vi "Read Thermocouples and Voltages v190401_A.vi"() -> ()   [LabVIEW 2017]
doc: "I. Description:\nThis example demonstrates how to make continuous, hardware-timed temperature measurement using a thermocouple.\n\nII. Instructions for Running:\n1. Specify the Physical Channel where you have connected the thermocouple.\n2. Enter the Minimum and Maximum temperature values in degrees C you expect to measure. A smaller range will allow a more accurate measurement.\n3. Enter the scan rate at which you want to run the acquisition.\n4. Specify the type of thermocouple you are using.\n5. Thermocouple measurements require cold-junction compensation (CJC) to correctly scale them. Specify the source of your cold-junction compensation.\n6. If your CJC source is \"Internal\", skip the rest of the steps.\n7. If your CJC source is \"Constant Value\", specify the value (usually room temperature) in degrees C.\n8. If your CJC source is \"Channel\", specify the CJC Channel name. \n9. Specify the appropriate Auto Zero Mode. See your device's hardware manual to find out if your device supports this attribute.\n\nIII. Block Diagram Steps:\n1. Create a Thermocouple (TC) temperature measurement channel.\n2. Get all the channels in the task.\n3. Convert channel(s) array to a comma-delimited channel string.\n4. This attribute is set to compensate for input offset errors. May not be supported by all devices*.\n5. Call the Timing VI to specify the hardware timing parameters. Use device's internal clock, continuous mode acquisition and the sample rate specified by the user.\n6. Call the Start VI to program and start the acquisition.\n7. Read N samples and plot it. By default, the Read VI reads all available samples, but you can specify how many samples to read at a time and the timeout value. Continue reading data until the stop button is pressed or an error occurs. \n8. Call the Clear Task VI to clear the Task.\n9. Use the popup dialog box to display an error if any.\n\n* If your device does not support Auto Zero Mode bypass Step 2, 3, and 4.\n\nIV. I/O Connections Overview:\nConnect your thermocouple to the terminals corresponding to the Physical Channel I/O Control value."
uses:
  <vilib>/Utility/error.llb/DialogType.ctl
  <vilib>/DAQmx/write.llb/DAQmx Write (Digital 1D Bool NChan 1Samp 1Line).vi
  <vilib>/DAQmx/read.llb/DAQmx Read (Analog 1D Wfm NChan NSamp).vi
  <vilib>/Analysis/baseanly.llb/Mean (DBL).vi
  <vilib>/DAQmx/create/channels.llb/DAQmx Create Channel (DO-Digital Output).vi
  <vilib>/Waveform/WDTOps.llb/WDT Index Channel DBL.vi
  <vilib>/DAQmx/create/channels.llb/DAQmx Create Channel (AI-Voltage-Basic).vi
  <vilib>/DAQmx/configure/timing.llb/DAQmx Timing (Sample Clock).vi
  <vilib>/DAQmx/miscellaneous.llb/DAQmx Fill In Error Info.vi
  <vilib>/express/express arith-compare/Formula/XNode/ExpressFormulaBlockNode.xnode
  <vilib>/Analysis/NI_AALBase.lvlib
  <vilib>/ptbypt/NI_PtbyPt.lvlib
  <vilib>/Utility/miscctls.llb/LVRowAndColumnTypeDef.ctl
panel:
  in  "Color Box":u32(colorbox)=16448250
  out "Micro-strain":dbl[](array[numeric]) format="%.2g"
  out "Results":i32[](listbox)
  in  "num_chans":i32=32
  in  "Search Strings":string[](array[string])=["Verbose Name", "Units", "Sensitivity", "Offset"]
  out "TRQ_2SPD_OT (N·m)":dbl=-0.01305389404296875 format="%0.3f"
  out "Power_OT (W)":dbl=-4.779110606064606 format="%.2f"
  out "rpm_out/rpm_in":dbl=-8.382425226893735e-05 format="%.3g"
  out "switch_counts":dbl=4500000.0
  in  "switch_time (s)":dbl=900000.0
  out "AI Consumer Iterations":i32=391128
  in  "LV_CMD_2SPD_OIL_SLND":bool[](array[boolean])=[FALSE]
  in  "lines":tag="Dev3/port1/line0"
  out "RPM_2SPD_OT_6602":dbl format="%0.1f"
  in  "path":path=path "N:/TeamShares/Testing Group/Bench Tests/PR22965 - Flow Test Magnum Lube Components/LabView Data"
  in  "DRVLN_PULLEY_RATIO":dbl=1.48 format="%.2f"
  out "P2 - P1":dbl=2.2560862731933593 format="%.3f"
  out "Recorded Blocks":dbl=295196.0
  out "AI Producer Iterations":i32=391127
  in  "Force Record":bool caption="Force Record Enable"
  out "RPM_DRVLN_6602":dbl format="%0.1f"
  out "data 2":waveform(dbl)[](array[waveform])=[{"t0"=timestamp(3621510319.1461306 s since 1904-01-01), "dt"=0.1, "Y"=[-0.0004730224609375, 0.00026397705078125], "attributes"=variant("NI_ChannelName"=variant(string "Dev1/ai0"), "NI_UnitDescription"=variant(string "Volts"))}, {"t0"=timestamp(3621510319.1461306 s since 1904-01-01), "dt"=0.1, "Y"=[1.0218643188476562, 1.0218521118164063], "attributes"=variant("NI_ChannelName"=variant(string "Dev1/ai0"), "NI_UnitDescription"=variant(string "Volts"))}, {"t0"=timestamp(3621510319.1461306 s since 1904-01-01), "dt"=0.1, "Y"=[1.5897842407226563, 1.5984542846679688], "attributes"=variant("NI_ChannelName"=variant(string "Dev1/ai0"), "NI_UnitDescription"=variant(string "Volts"))}, {"t0"=timestamp(3621510319.1461306 s since 1904-01-01), "dt"=0.1, "Y"=[1.525469970703125, 1.533917236328125], "attributes"=variant("NI_ChannelName"=variant(string "Dev1/ai0"), "NI_UnitDescription"=variant(string "Volts"))}, {"t0"=timestamp(3621510319.1461306 s since 1904-01-01), "dt"=0.1, "Y"=[3.0046722412109377, 3.0046966552734373], "attributes"=variant("NI_ChannelName"=variant(string "Dev1/ai0"), "NI_UnitDescription"=variant(string "Volts"))}, {"t0"=timestamp(3621510319.1461306 s since 1904-01-01), "dt"=0.1, "Y"=[1.769482421875, 1.7677413940429687], "attributes"=variant("NI_ChannelName"=variant(string "Dev1/ai0"), "NI_UnitDescription"=variant(string "Volts"))}, {"t0"=timestamp(3621510319.1461306 s since 1904-01-01), "dt"=0.1, "Y"=[-0.0179168701171875, -0.0179443359375], "attributes"=variant("NI_ChannelName"=variant(string "Dev1/ai0"), "NI_UnitDescription"=variant(string "Volts"))}, {"t0"=timestamp(3621510319.1461306 s since 1904-01-01), "dt"=0.1, "Y"=[-0.0014312744140625, -0.00116424560546875], "attributes"=variant("NI_ChannelName"=variant(string "Dev1/ai0"), "NI_UnitDescription"=variant(string "Volts"))}, {"t0"=timestamp(3621510319.1461306 s since 1904-01-01), "dt"=0.1, "Y"=[-0.00082550048828125, -0.0017852783203125], "attributes"=variant("NI_ChannelName"=variant(string "Dev1/ai0"), "NI_UnitDescription"=variant(string "Volts"))}, {"t0"=timestamp(3621510319.1461306 s since 1904-01-01), "dt"=0.1, "Y"=[2.997636413574219, 2.9961593627929686], "attributes"=variant("NI_ChannelName"=variant(string "Dev1/ai0"), "NI_UnitDescription"=variant(string "Volts"))}, {"t0"=timestamp(3621510319.1461306 s since 1904-01-01), "dt"=0.1, "Y"=[-1.52587890625e-05, -0.00017242431640625], "attributes"=variant("NI_ChannelName"=variant(string "Dev1/ai0"), "NI_UnitDescription"=variant(string "Volts"))}, {"t0"=timestamp(3621510319.1461306 s since 1904-01-01), "dt"=0.1, "Y"=[0.002484130859375, 0.00252532958984375], "attributes"=variant("NI_ChannelName"=variant(string "Dev1/ai0"), "NI_UnitDescription"=variant(string "Volts"))}, {"t0"=timestamp(3621510319.1461306 s since 1904-01-01), "dt"=0.1, "Y"=[-0.10861358642578126, -0.10858306884765626], "attributes"=variant("NI_ChannelName"=variant(string "Dev1/ai0"), "NI_UnitDescription"=variant(string "Volts"))}, {"t0"=timestamp(3621510319.1461306 s since 1904-01-01), "dt"=0.1, "Y"=[-1.1660736083984375, -1.1659881591796875], "attributes"=variant("NI_ChannelName"=variant(string "Dev1/ai0"), "NI_UnitDescription"=variant(string "Volts"))}, {"t0"=timestamp(3621510319.1461306 s since 1904-01-01), "dt"=0.1, "Y"=[-1.0824356079101562, -1.0823379516601563], "attributes"=variant("NI_ChannelName"=variant(string "Dev1/ai0"), "NI_UnitDescription"=variant(string "Volts"))}, {"t0"=timestamp(3621510319.1461306 s since 1904-01-01), "dt"=0.1, "Y"=[-0.1474090576171875, -0.14737548828125], "attributes"=variant("NI_ChannelName"=variant(string "Dev1/ai0"), "NI_UnitDescription"=variant(string "Volts"))}]
  out "Power_IN (W)":dbl=0.0005711775684961294 format="%.2g"
  out "TRQ_2SPD_DRVLN_OT (N·m)":dbl=-0.018612060546874976 format="%0.3f"
  out "Waveform Chart":waveform(dbl)[](graph)=[{"t0"=timestamp(3634059218.103555 s since 1904-01-01), "dt"=0.1, "Y"=[0.0040825469970704464, 0.004508938598632994], "attributes"=variant("NI_ChannelName"=variant(string "P1_OIL_FILTER_OT"), "NI_UnitDescription"=variant(string "bar g"))}, {"t0"=timestamp(3634059218.103555 s since 1904-01-01), "dt"=0.1, "Y"=[2.0849262466430662, 2.0811629058837893], "attributes"=variant("NI_ChannelName"=variant(string "P2_OIL_PUMP_CTRL"), "NI_UnitDescription"=variant(string "bar g"))}, {"t0"=timestamp(3634059218.103555 s since 1904-01-01), "dt"=0.1, "Y"=[2.0002626892089843, 1.9966154815673829], "attributes"=variant("NI_ChannelName"=variant(string "P3_OIL_PUMP_OT"), "NI_UnitDescription"=variant(string "bar g"))}, {"t0"=timestamp(3634059218.103555 s since 1904-01-01), "dt"=0.1, "Y"=[-11.107454470825196, -11.112982447814943], "attributes"=variant("NI_ChannelName"=variant(string "P4_OIL_LUBE_OT"), "NI_UnitDescription"=variant(string "bar g"))}, {"t0"=timestamp(3634059218.103555 s since 1904-01-01), "dt"=0.1, "Y"=[-2.105040821838379, -2.1068857055664063], "attributes"=variant("NI_ChannelName"=variant(string "P5_SPARE"), "NI_UnitDescription"=variant(string "bar g"))}, {"t0"=timestamp(3634059218.103555 s since 1904-01-01), "dt"=0.1, "Y"=[-3.1523495605468748, -3.15418076171875], "attributes"=variant("NI_ChannelName"=variant(string "P6_SPARE"), "NI_UnitDescription"=variant(string "bar g"))}, {"t0"=timestamp(3634059218.103555 s since 1904-01-01), "dt"=0.1, "Y"=[-0.927960205078125, -0.9276962280273438], "attributes"=variant("NI_ChannelName"=variant(string "P7_SPARE"), "NI_UnitDescription"=variant(string "bar a"))}, {"t0"=timestamp(3634059218.103555 s since 1904-01-01), "dt"=0.1, "Y"=[0.02285817565917947, 0.02207293701171853], "attributes"=variant("NI_ChannelName"=variant(string "P8_OIL_COOLER_OT"), "NI_UnitDescription"=variant(string "bar g"))}, {"t0"=timestamp(3634059218.103555 s since 1904-01-01), "dt"=0.1, "Y"=[1410.0847681655885, 1409.1728451538086], "attributes"=variant("NI_ChannelName"=variant(string "RPM_2SPD_IN_FV"), "NI_UnitDescription"=variant(string "RPM"))}, {"t0"=timestamp(3634059218.103555 s since 1904-01-01), "dt"=0.1, "Y"=[1374.9208407257079, 1374.7411578094482], "attributes"=variant("NI_ChannelName"=variant(string "RPM_2SPD_OT_FV"), "NI_UnitDescription"=variant(string "RPM"))}, {"t0"=timestamp(3634059218.103555 s since 1904-01-01), "dt"=0.1, "Y"=[51.3275146484375, 51.390533447265625], "attributes"=variant("NI_ChannelName"=variant(string "T_OIL_PUMP_OT"), "NI_UnitDescription"=variant(string "°C"))}, {"t0"=timestamp(3634059218.103555 s since 1904-01-01), "dt"=0.1, "Y"=[69.04945373535156, 69.14482116699219], "attributes"=variant("NI_ChannelName"=variant(string "T_OIL_SPARE"), "NI_UnitDescription"=variant(string "°C"))}, {"t0"=timestamp(3634059218.103555 s since 1904-01-01), "dt"=0.1, "Y"=[-4.136749267578125, -4.28717041015625], "attributes"=variant("NI_ChannelName"=variant(string "TRQ_PMP_IN"), "NI_UnitDescription"=variant(string "N·m"))}, {"t0"=timestamp(3634059218.103555 s since 1904-01-01), "dt"=0.1, "Y"=[-0.009429931640625, -0.0040740966796875], "attributes"=variant("NI_ChannelName"=variant(string "TRQ_2SPD_OT"), "NI_UnitDescription"=variant(string "N·m"))}, {"t0"=timestamp(3634059218.103555 s since 1904-01-01), "dt"=0.1, "Y"=[0.22497978210449232, 0.2247674942016602], "attributes"=variant("NI_ChannelName"=variant(string "VFr_660_0380_OT"), "NI_UnitDescription"=variant(string "gpm"))}, {"t0"=timestamp(3634059218.103555 s since 1904-01-01), "dt"=0.1, "Y"=[-14.992698669433594, -14.993682861328125], "attributes"=variant("NI_ChannelName"=variant(string "VFr_OIL_LUBE_OT"), "NI_UnitDescription"=variant(string "gpm"))}, {"t0"=timestamp(3634059218.103555 s since 1904-01-01), "dt"=0.1, "Y"=[1.48, 1.48], "attributes"=variant("NI_ChannelName"=variant(string "RPM_RATIO"), "NI_UnitDescription"=variant(string "ratio"))}, {"t0"=timestamp(3634059218.103555 s since 1904-01-01), "dt"=0.1, "Y"=[99.0, 99.0], "attributes"=variant("NI_ChannelName"=variant(string "DataTag"), "NI_UnitDescription"=variant(string "none"))}, {"t0"=timestamp(3634059218.103555 s since 1904-01-01), "dt"=0.1, "Y"=[0.0, 0.0], "attributes"=variant("NI_ChannelName"=variant(string "LV_CMD_2SPD_OIL_SLND"), "NI_UnitDescription"=variant(string "boolean"))}]
  in  "Run Letter":string="a"
  out "Recording":bool
  in  "Num_Blocks":dbl=100.0
  in  "Data Tag":dbl=99.0 format="%.2p"
  in  "Maximum Value":dbl=10.0 format="%0.2f"
  in  "Minimum Value":dbl=-10.0 format="%0.2f"
  in  "Physical Channel":tag="Dev4/ai0:31" caption="PCI-6143_1 Channels"
  in  "stop":bool
  in  "Rate":dbl=1000.0 format="%0.2f"
  # "rev 150415_A  added \"Record Run X\" sub VI.\nrev 150423_A added power, efficiency, and manual inputs for speed .\nrev 150423_B added speed measurement via PCI-6602 card.\nrev 161117_A is set up for the alternator test reading shaft RPM from Dynapar encoder and torque from the Omega TQ513-1K paired with the Omega DP41-S.\nrev 170504_A migrated DAQ h/w from the SCXI chassis (now being used for TC2 porcupine testing) to PCI-6143.\nrev 170510_A takes data at 1000Hz, then averages groups of 100 samples for a logging rate of 10Hz per channel.  Added function that resets \"Data Tag\"\nto 99 after \"Num_Blocks\" has been recorded.\nrev 170810_A adds flowmeter for 2-speed supercharger drive bench test.  CJP\nrev 170821_A logs tags to same file for a given run letter.  Uses \"Record Continuous Tags...\" sub VI.\nrev 171129_A is for the Orthrus 2-speed drive.  Added new encoder period measurement for the 127 tooth geat \"RPM_2SPD_OT\". CJP\nrev 171130_A adds Digital Output (DO) for 2SPD drive control.  Will log this with the rest of the data.  Also corrected the number of teeth on the 2SPD Output side from 127 to 107!\nrev 171201_A restructuring for  \"real-time\" response to speed changes by moving the disklog to a separate loop (queue).\nrev 171201_B moves counters into main AI loop and adds a start trigger so DAQ won't start until rig is spinning.  Added F-V where old \"F1\" channel was for \"RPM_2SPD_OT\".   CJP\nrev 171201_C uses a CI-Frequency task for RPM instead of period.  Testing this for better transient response.  This appears to be even slower than the period measurement.\nrev 171201_D is built from rev 171201_A, but adding in the F-V channel.  This version queues both the AI channel and CI channels to a single Consumer.  Also adding a 30s switch to automate switching of the 2SPD solenoid.\nrev 171221_A was the first attempt at this and for some reason, while running that VI, the computer froze, unable to do ctrl+alt+del reboot.  After rebooting, the VI was no longer openable in LabView 2014 or LabView 2016.  Will try the same process over with v171226_A.\nrev 171226_A adds one more PCI_6143 card for 8 additional analog inputs.\nrev 171226_B created a backup with 171226_A.\nrev 180314_A added thermocouple for Sumanth.  This is for testing the 2-Speed Drive.\nrev Read \"ThermVolt_TestSpeed_180406_A.vi\" is for verifying the one remaining Micro-Epsilon speed sensor on the 2Spd Drive.\nrev \"Read Thermocouples and Voltages v180406_A.vi\" reintroduces the two counter/timer channels on the PCI-6602 card for the driveline encoder and \nMicro-Epsilon 2Spd Output.\nrev 180919_A built off of rev 180426_A for 2-Speed Drive testing.  CJP\nv181002_A adding new T22 at 2SPD input pulley AND keeping original T22 at output end of drivline.  CJP\nv181004_A corrected front panel displays for Power_IN and Power_OT.  CJP\nv181025_A adding ReadChnCfg.VI to read channel names, units, scaling, and offset from Labview Channel Map\nv190401_A restructuring \"Read Thermocouples and Voltages...\" to use only channels from NI-6229 out of test cell 2.  CJP"
  # "For instructions, select Help>>Show Context Help"
  # "Now using 360 PPR encoder for input speed 171227.\nChanged to Input Gear Speed 180118.  CJP  127 Hz = 1 RPS, 127 Hz = 60 RPM\n5 kHz = 1 V => 5000/127 = 39.37 RPS = 2362.205 RPM\nv180314_A 5kHz = 1V = 5000/360 = 13.888 RPS = 833.33 RPM.\nBack to 360PPR encoder with pulley ratio of 1.48."
  # "HBM T21WN"
  # "Interface T22"
  # "Timing Parameters"
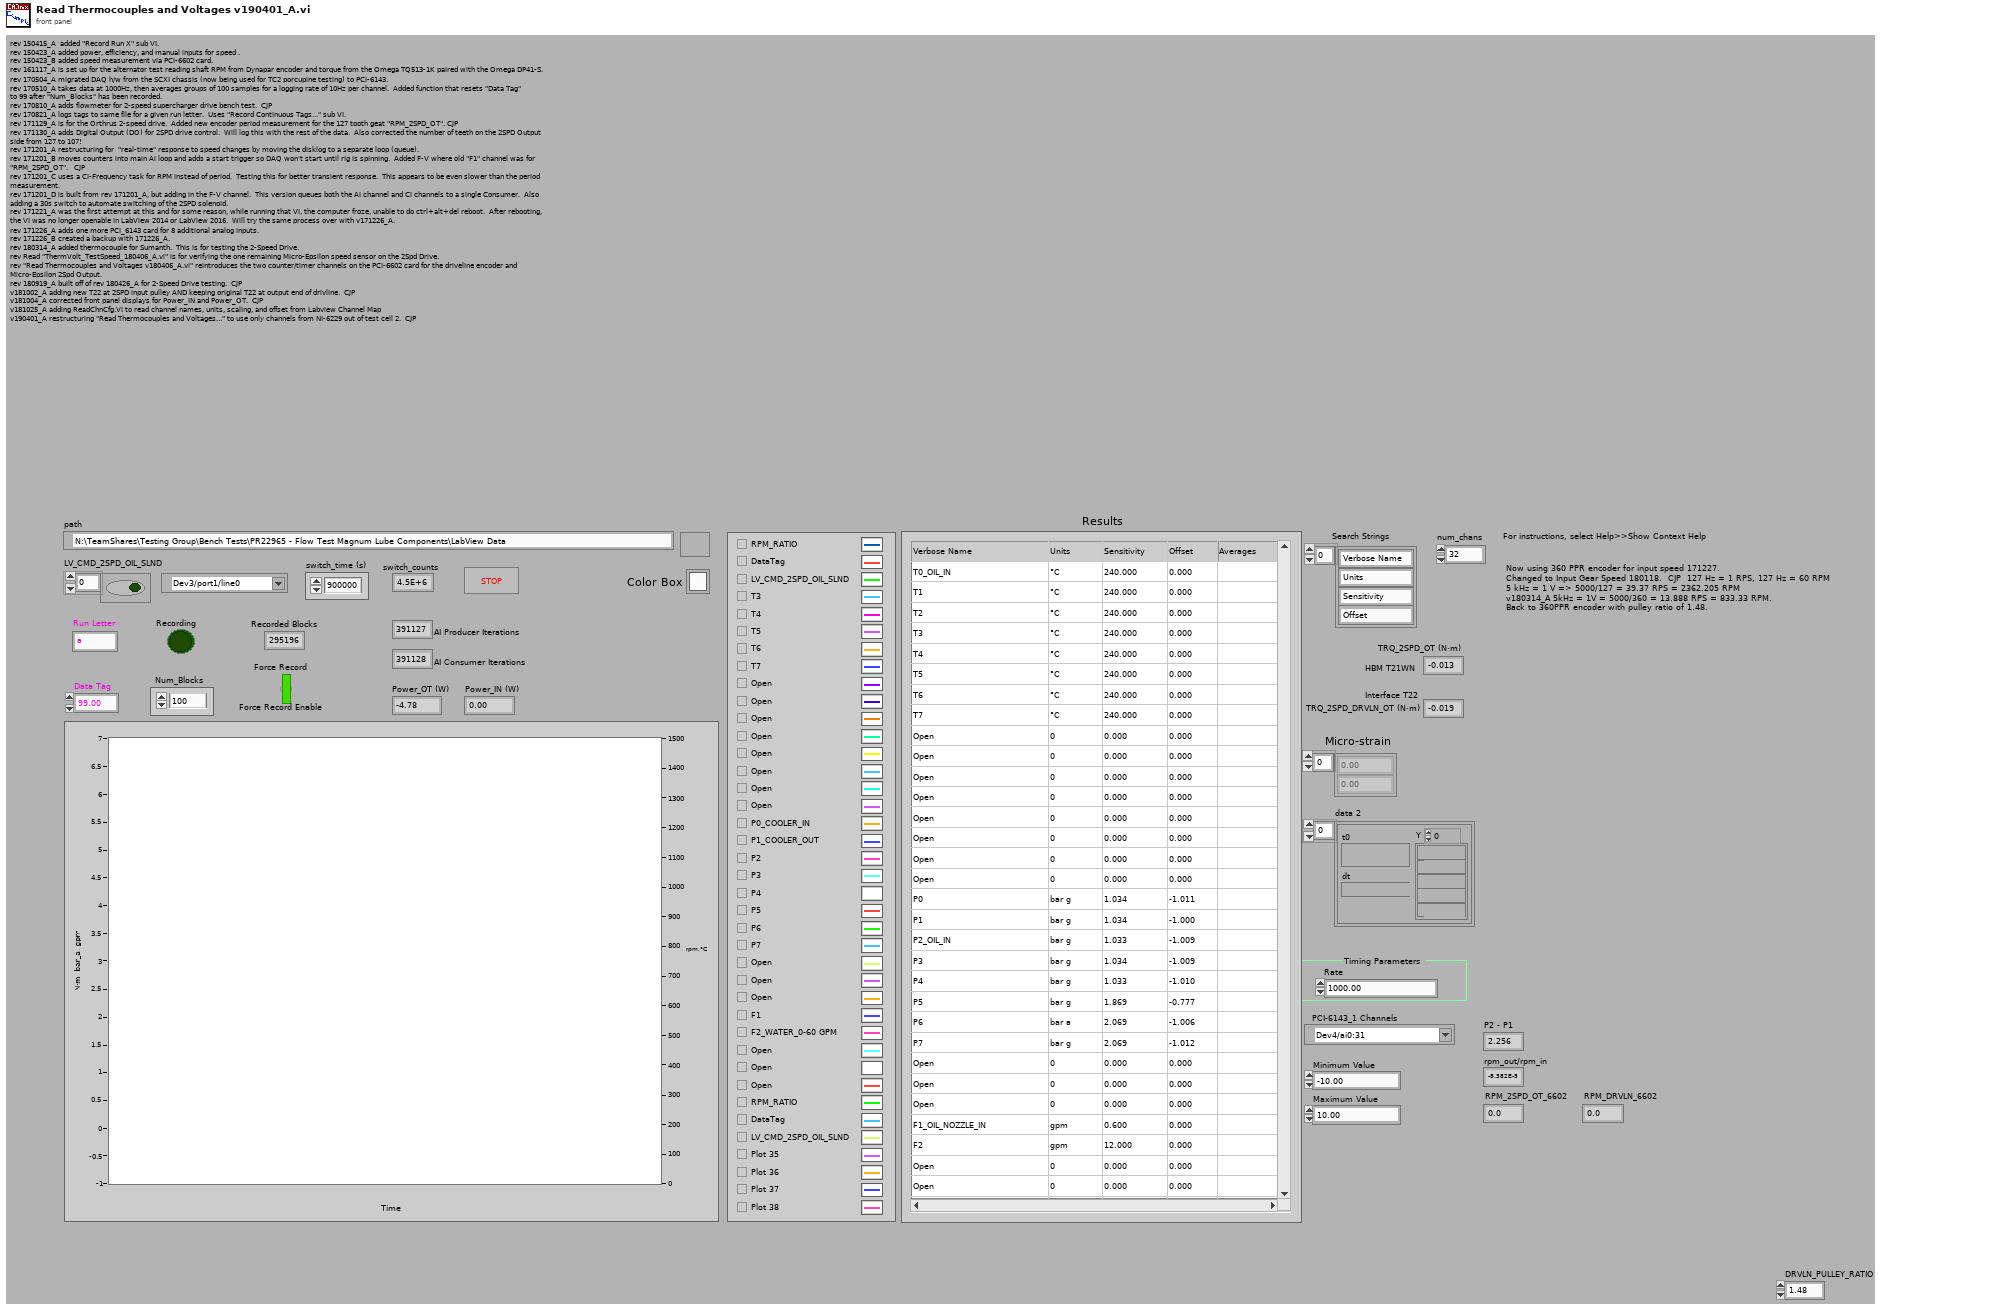
[diagram p1: front panel]
types:
  T1 = typedef "DialogType.ctl" = u16
  T2 = typedef "LVRowAndColumnTypeDef.ctl" = cluster{"Row":i32, "Column":i32}
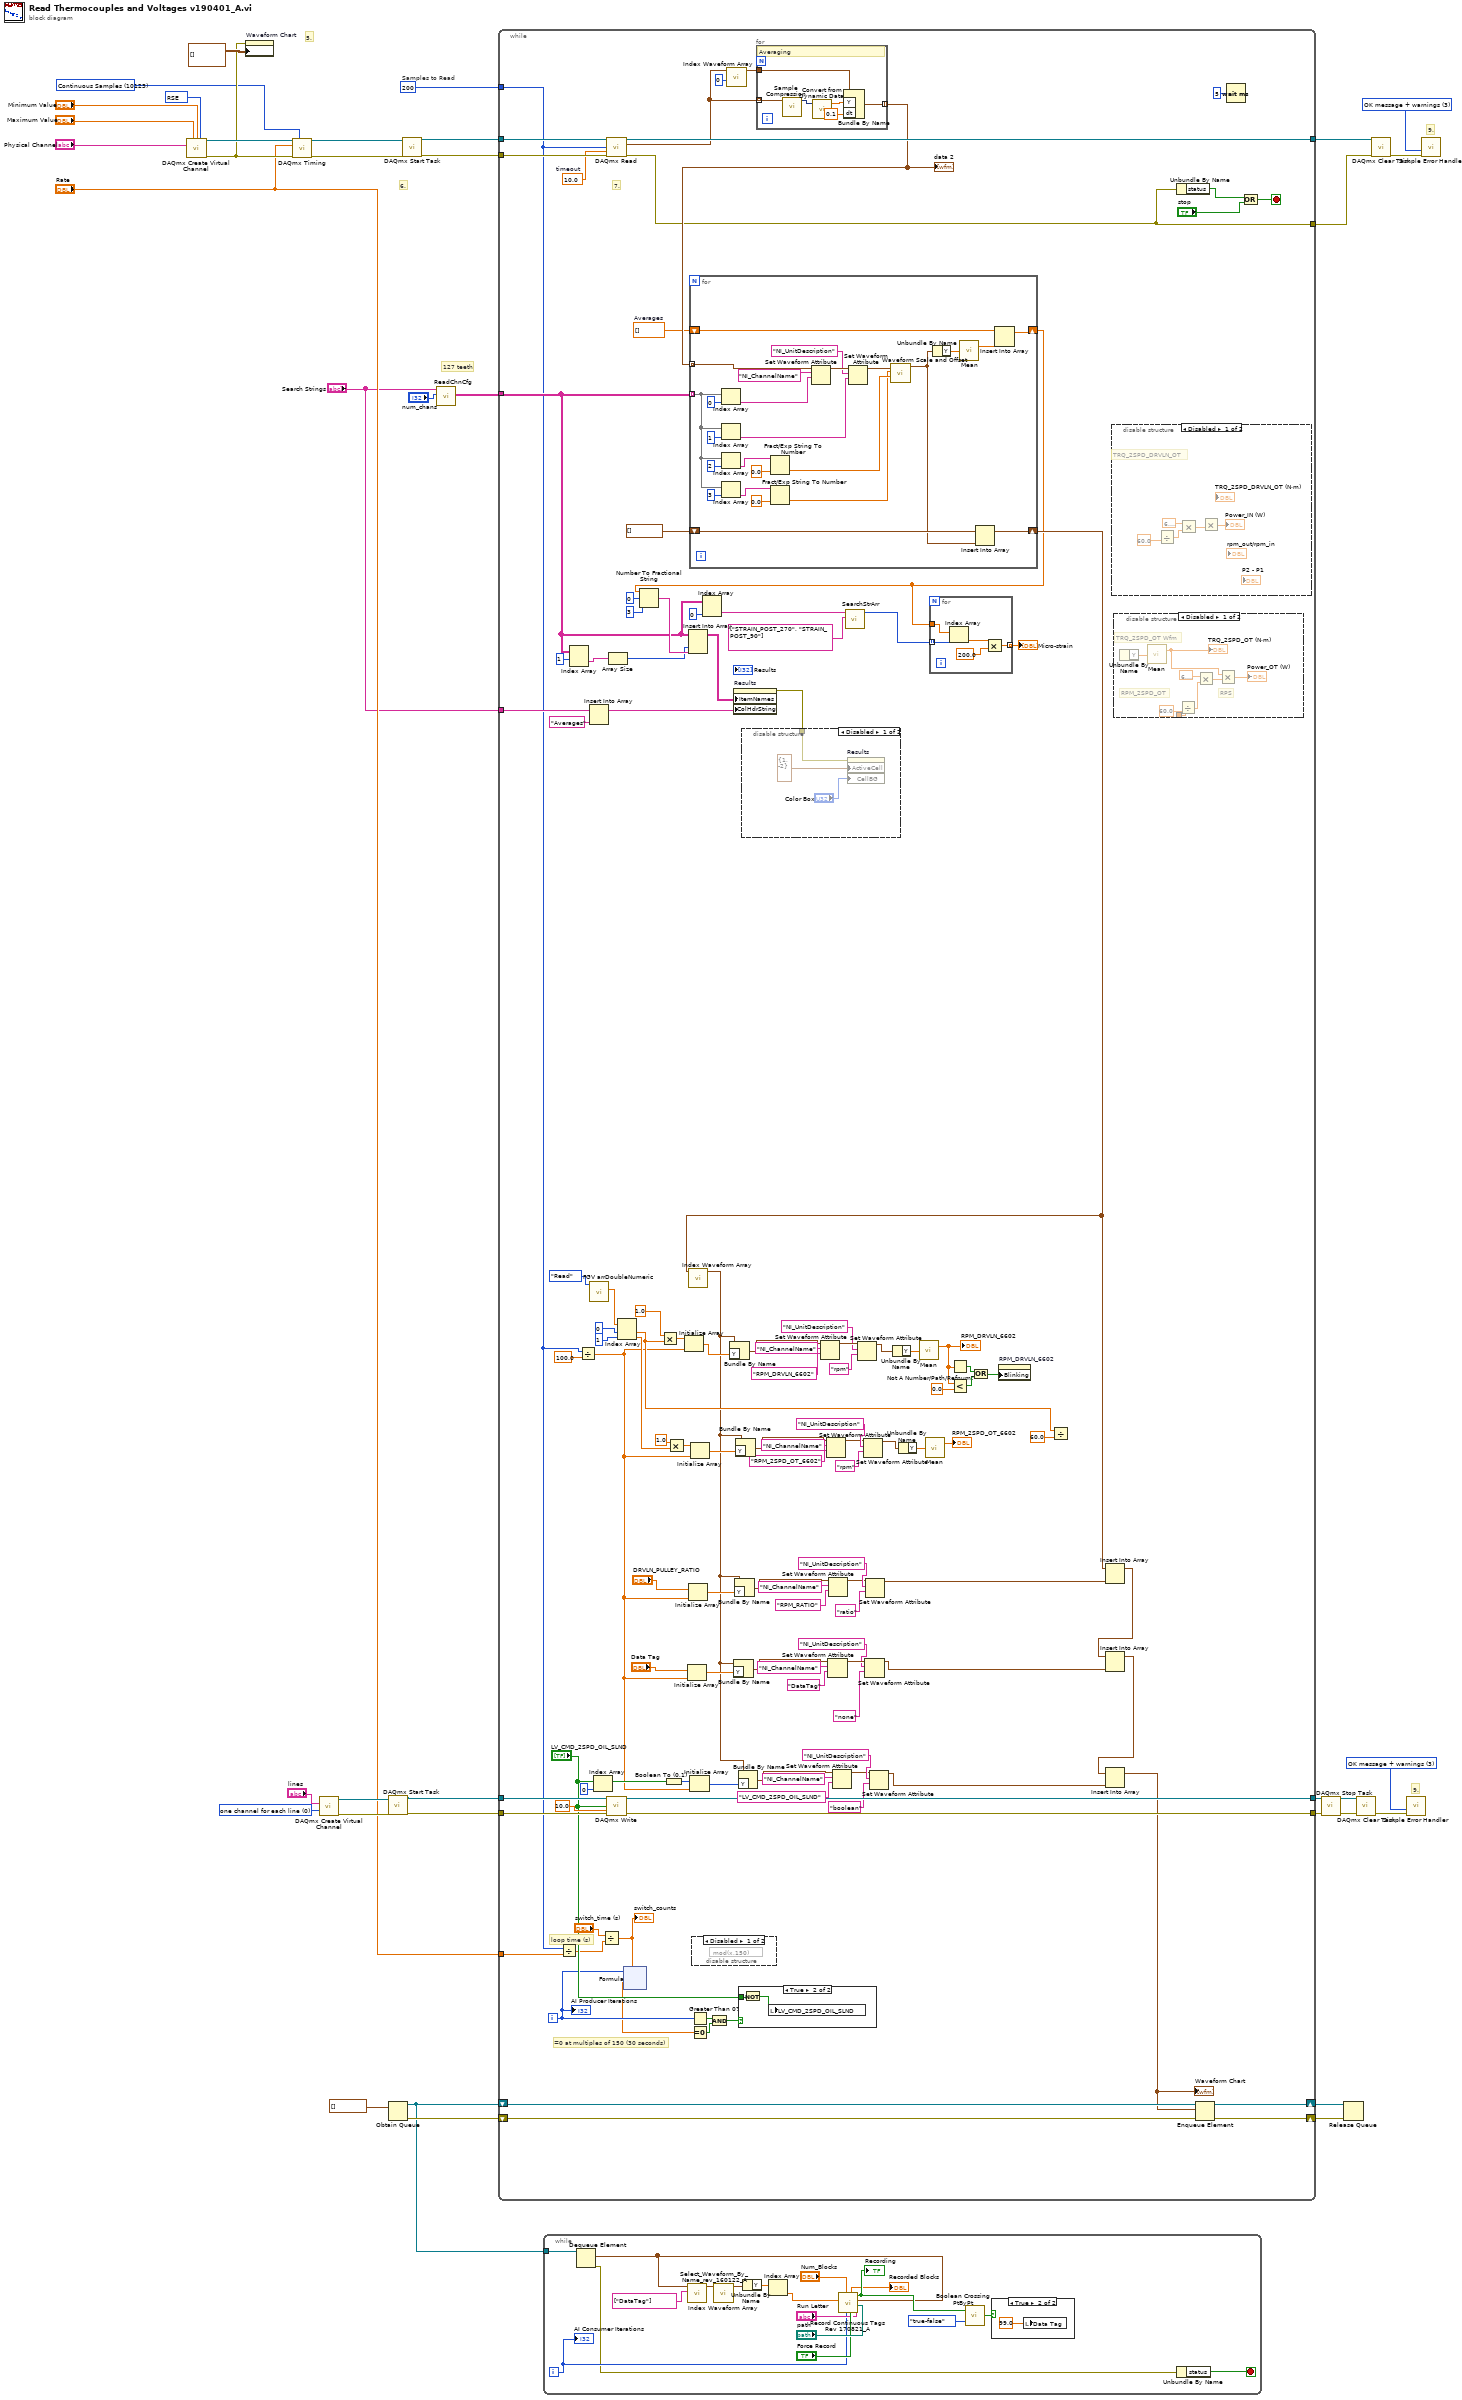
[diagram p0: block diagram]
diagram:
  w1 = 10083 items=["Default"=-1, "RSE"=10083, "NRSE"=10078, "Differential"=10106, "Pseudodifferential"=12529] ("input terminal configuration")
  w21 = T1 3 items=["no dialog", "OK message", "continue or stop message", "OK message + warnings", "continue/stop + warnings"] ("type of dialog (OK msg:1)")
  w27 = 0 items=["one channel for each line", "one channel for all lines"] ("line grouping")
  w33 = T1 3 items=["no dialog", "OK message", "continue or stop message", "OK message + warnings", "continue/stop + warnings"] ("type of dialog (OK msg:1)")
  w7 = 10123 items=["Finite Samples"=10178, "Continuous Samples"=10123] ("sample mode")
  # "127 teeth"
  # "Samples to Read"
  # "9."
  # "9."
  # "5."
  # "6."
  n1 = call-poly <vilib>:"DAQmx Create Virtual Channel.vi"("maximum value"="Maximum Value", "minimum value"="Minimum Value", "input terminal configuration"=w1, "physical channels"="Physical Channel") -> ("task out"=w31:refnum<k21>, "error out"=w29:errorcluster)  [unwired: 10 in]
  n2 = property on="Waveform Chart" class="WFChart (strict)"(error in=w29, "History Data"=waveform(dbl)[][] []) -> ()  [unwired: 1 in, 2 out]
  n3 = call-poly <vilib>:"DAQmx Timing.vi"("task/channels in"=w31, "sample mode"=w7, "rate"="Rate", "error in"=w29) -> ("task out"=w34:refnum<k21>, "error out"=w2:errorcluster)  [unwired: 10 in]
  n4 = call-poly <vilib>:"DAQmx Create Virtual Channel.vi"("lines"="lines", "line grouping"=w27) -> ("task out"=w26:refnum<k21>, "error out"=w25:errorcluster)  [unwired: 12 in]
  n5 = call <vilib>:"DAQmx Start Task.vi"("task/channels in"=w26, "error in"=w25) -> ("task out"=w24:refnum<k21>, "error out"=w23:errorcluster)  [unwired: 12 in]
  n6 = Obtain Queue(element data type=waveform(dbl)[] [] ("appended array")) -> (queue out=w11:refnum<queue>, error out=w14:errorcluster)  [unwired: 4 in, 1 out]
  n7 = call <vilib>:"DAQmx Start Task.vi"("task/channels in"=w34, "error in"=w2) -> ("task out"=w36:refnum<k21>, "error out"=w37:errorcluster)  [unwired: 12 in]
  n8 = call "ReadChnCfg.vi"("num_chans"="num_chans", "Search Strings"="Search Strings") -> ("Table Minus Headers"=w5:string[][])  [unwired: 8 in, 1 out]
  n9 = while {
    tunnel: w36 -> [w162]
    tunnel: w37 -> [w161]
    tunnel: [w160] -> w35
    tunnel: 200 ("number of samples per channel") -> [w40]
    tunnel: w24 -> [w106]
    tunnel: w23 -> [w105]
    tunnel: [w104] -> w18
    tunnel: [w103] -> w17
    shift-right: [w89] -> w13
    shift-left: w11 -> [w91]
    shift-right: [w88] -> w12
    shift-left: w14 -> [w90]
    tunnel: "Rate" -> [w82]
    tunnel: [w42] -> w3
    tunnel: w5 -> [w49]
    tunnel: "Search Strings" -> [w59]
    i -> [w79]
    stop <- w157 stop-if-true
    w70 = dbl[] []  # Averages
    w158 = 10.0  # timeout
    # "loop time (s)"
    # "=0 at multiples of 150 (30 seconds)"
    # "7."
    n10 = Divide(x=w40, y=w82) -> (x/y=w81:dbl)
    n11 = Index Array(array=w49, index (row)=1) -> (element=w53:string[])  [unwired: 1 in]
    n12 = Divide(x=w40, y=100.0) -> (x/y=w92:dbl)
    n13 = Insert Into Array(array=w59, new element="Averages" ("new element/subarray")) -> (w50:string[])  [unwired: 1 in]
    n14 = call "FGV arrDoubleNumeric.vi"("Enum"=enum16{"Read", "Write"}."Read") -> ("Array OUT"=w121:dbl[])  [unwired: 9 in, 1 out]
    n15 = Index Array(array="LV_CMD_2SPD_OIL_SLND", index=0) -> (element=w100:bool)
    n16 = Divide(x="switch_time (s)", y=w81) -> (x/y=w78:dbl)
    "switch_counts" <- w78
    n17 = call-poly <vilib>:"DAQmx Read.vi"("task/channels in"=w162, "number of samples per channel"=w40, "timeout"=w158, "error in"=w161) -> ("task out"=w160:refnum<k21>, "data"=w41:waveform(dbl)[], "error out"=w42:errorcluster)  [unwired: 9 in]
    n18 = call-poly <vilib>:"DAQmx Write.vi"("task/channels in"=w106, "data"="LV_CMD_2SPD_OIL_SLND", "timeout"=10.0, "error in"=w105) -> ("task out"=w104:refnum<k21>, "error out"=w103:errorcluster)  [unwired: 9 in, 1 out]
    n19 = Array Size(array=w53) -> (size(s)=w52:i32)
    n20 = Index Array(array=w121, index #1=0 ("index"), index #2=1 ("index")) -> (element #1=w120:dbl, element #2=w107:dbl)
    n21 = xnode "Formula"("X1"=w79, "X2"=w78) -> ("Result"=w77:dbl)  [unwired: 1 in, 1 out]
    n22 = Multiply(x=1.0, y=w120) -> (x*y=w138:dbl)
    n23 = Boolean To (0,1)(Boolean=w100) -> (0, 1=w93:i16)
    n24 = Multiply(x=1.0, y=w107) -> (x*y=w115:dbl)
    n25 = Initialize Array(w138, w92) -> (w146:dbl[])
    n26 = Initialize Array("Data Tag", w92) -> (w123:dbl[])
    n27 = Initialize Array("DRVLN_PULLEY_RATIO", w92) -> (w136:dbl[])
    n28 = Initialize Array(w93, w92) -> (w87:i16[])
    n29 = Initialize Array(w115, w92) -> (w114:dbl[])
    n30 = Greater Than 0?(x=w79) -> (x > 0?=w84:bool)
    n31 = Equal To 0?(x=w77) -> (x = 0?=w83:bool)
    n32 = disable-structure shown="Disabled" {
      frame Disabled {
        n33 = expression code="mod(x,150)"() -> ()  [unwired: 1 in, 1 out]
      }
      frame Enabled {
      }
    }
    n34 = Index Array(array=w49, index (col)=0 ("disabled index (col)")) -> (element=w47:string[])  [unwired: 1 in]
    n35 = And(x=w84, y=w83) -> (x .and. y?=w85:bool)
    n36 = call-poly <vilib>:"Index Waveform Array.vi"("index"=0, "waveform array"=w41) -> ("waveform"=w139:waveform(dbl))  [unwired: 8 in, 1 out]
    n37 = case shown="True" w85 {
      tunnel: "LV_CMD_2SPD_OIL_SLND" -> [_ w220]
      frame False {
      }
      frame True {
        n38 = Not(x=w220) -> (.not. x?=w219:bool[])
        n39 = local write "LV_CMD_2SPD_OIL_SLND"(w219) -> ()
      }
    }
    n40 = for {
      tunnel: w41 -> [w223] mode=indexing
      tunnel: [w222] -> w72 mode=indexing
      tunnel: w139 -> [w221]
      # "Averaging"
      n41 = call "Sample Compression"("Signals"=w223) -> ("Mean"=w224:dynamicdata)  [unwired: 8 in, 2 out]
      n42 = call "Convert from Dynamic Data"("Dynamic Data Type"=w224) -> ("Array"=w226:dbl[])  [unwired: 3 in]
      n43 = Bundle By Name(cluster=w221, "Y"=w226, "dt"=0.1) -> (w222:waveform(dbl))
    }
    "data 2" <- w72
    n44 = for {
      tunnel: w72 -> [w195] mode=indexing
      shift-right: [w194] -> w44
      shift-left: w70 -> [w193]
      tunnel: w49 -> [w182] mode=indexing
      shift-right: [w189] -> w66
      shift-left: waveform(dbl)[] [] -> [w191]
      n45 = Index Array(array=w182, index=0) -> (element=w186:string)
      n46 = Index Array(array=w182, index=1) -> (element=w185:string)
      n47 = Index Array(array=w182, index=2) -> (element=w181:string)
      n48 = Index Array(array=w182, index=3) -> (element=w177:string)
      n49 = Fract/Exp String To Number(string=w181, default (0 dbl)=0.0) -> (number=w179:dbl)  [unwired: 2 in, 1 out]
      n50 = Fract/Exp String To Number(string=w177, default (0 dbl)=0.0) -> (number=w176:dbl)  [unwired: 2 in, 1 out]
      n51 = Set Waveform Attribute(5:w186, 6:"NI_ChannelName" ("name"), 7:w195) -> (3:w199:waveform(dbl))  [unwired: 1 in, 2 out]
      n52 = Set Waveform Attribute(5:w185, 6:"NI_UnitDescription" ("name"), 7:w199) -> (3:w197:waveform(dbl))  [unwired: 1 in, 2 out]
      n53 = call <vilib>:"Waveform Scale and Offset.vi"("scale"=w179, "offset"=w176, "waveform in"=w197) -> ("waveform out"=w190:waveform(dbl))  [unwired: 7 in, 1 out]
      n54 = Unbundle By Name(w190) -> ("Y"=w196:dbl[])
      n55 = call-poly <vilib>:"Mean.vi"("X"=w196) -> ("mean"=w192:dbl)  [unwired: 1 out]
      n56 = Insert Into Array(array=w191, new element=w190) -> (w189:waveform(dbl)[])  [unwired: 1 in]
      n57 = Insert Into Array(array=w193, new element=w192) -> (w194:dbl[])  [unwired: 1 in]
    }
    n58 = Number To Fractional String(number=w44, width (-)=i16 0, precision (6)=i16 3) -> (F-format string=w55:string[])  [unwired: 1 in]
    n59 = Insert Into Array(array=w49, index (col)=w52, new element=w55) -> (w51:string[][])  [unwired: 1 in]
    n60 = call-poly <vilib>:"Index Waveform Array.vi"("waveform array"=w66) -> ("waveform"=w67:waveform(dbl))  [unwired: 9 in, 1 out]
    n61 = Bundle By Name(cluster=w67, "Y"=w146) -> (w137:waveform(dbl))
    n62 = property on="Results" class="MCListbox (strict)"("ItemNames"=w51, "ColHdrString"=w50) -> (error out=w39:errorcluster)  [unwired: 2 in, 1 out]
    n63 = Bundle By Name(cluster=w67, "Y"=w123) -> (w129:waveform(dbl))
    n64 = Bundle By Name(cluster=w67, "Y"=w136) -> (w130:waveform(dbl))
    n65 = Bundle By Name(cluster=w67, "Y"=w114) -> (w116:waveform(dbl))
    n66 = Bundle By Name(cluster=w67, "Y"=w87) -> (w94:waveform(dbl))
    n67 = disable-structure shown="Disabled" {
      disable-tunnel: w39 -> [w165 _]
      frame Disabled {
        n68 = property on="Results" class="MCListbox (strict)"(error in=w165, "ActiveCell"=T2 {"Row"=1, "Column"=-2} ("Active Cell:Active Cell"), "CellBG"="Color Box") -> ()  [unwired: 1 in, 2 out]
      }
      frame Enabled {
      }
    }
    n69 = Set Waveform Attribute(5:"RPM_DRVLN_6602" ("name"), 6:"NI_ChannelName" ("name"), 7:w137) -> (3:w150:waveform(dbl))  [unwired: 1 in, 2 out]
    n70 = Set Waveform Attribute(5:"RPM_2SPD_OT_6602" ("name"), 6:"NI_ChannelName" ("name"), 7:w116) -> (3:w110:waveform(dbl))  [unwired: 1 in, 2 out]
    n71 = Set Waveform Attribute(5:"DataTag" ("name"), 6:"NI_ChannelName" ("name"), 7:w129) -> (3:w127:waveform(dbl))  [unwired: 1 in, 2 out]
    n72 = Set Waveform Attribute(5:"RPM_RATIO" ("name"), 6:"NI_ChannelName" ("name"), 7:w130) -> (3:w132:waveform(dbl))  [unwired: 1 in, 2 out]
    n73 = Set Waveform Attribute(5:"LV_CMD_2SPD_OIL_SLND" ("name"), 6:"NI_ChannelName" ("name"), 7:w94) -> (3:w96:waveform(dbl))  [unwired: 1 in, 2 out]
    n74 = call "SearchStrArr.vi"("asSearchList"=string[] ["STRAIN_POST_270", "STRAIN_POST_90"], "asDict"=w47) -> ("aiRowIdx"=w45:i32[])  [unwired: 9 in]
    n75 = Set Waveform Attribute(5:"rpm" ("name"), 6:"NI_UnitDescription" ("name"), 7:w150) -> (3:w68:waveform(dbl))  [unwired: 1 in, 2 out]
    n76 = Set Waveform Attribute(5:"rpm" ("name"), 6:"NI_UnitDescription" ("name"), 7:w110) -> (3:w73:waveform(dbl))  [unwired: 1 in, 2 out]
    n77 = Set Waveform Attribute(5:"none" ("name"), 6:"NI_UnitDescription" ("name"), 7:w127) -> (3:w61:waveform(dbl))  [unwired: 1 in, 2 out]
    n78 = Set Waveform Attribute(5:"ratio" ("name"), 6:"NI_UnitDescription" ("name"), 7:w132) -> (3:w65:waveform(dbl))  [unwired: 1 in, 2 out]
    n79 = Set Waveform Attribute(5:"boolean" ("name"), 6:"NI_UnitDescription" ("name"), 7:w96) -> (3:w60:waveform(dbl))  [unwired: 1 in, 2 out]
    n80 = Unbundle By Name(w68) -> ("Y"=w147:dbl[])
    n81 = Unbundle By Name(w73) -> ("Y"=w113:dbl[])
    n82 = call-poly <vilib>:"Mean.vi"("X"=w147) -> ("mean"=w75:dbl)  [unwired: 1 out]
    "RPM_DRVLN_6602" <- w75
    n83 = call-poly <vilib>:"Mean.vi"("X"=w113) -> ("mean"=→"RPM_2SPD_OT_6602":dbl)  [unwired: 1 out]
    n84 = for {
      tunnel: w45 -> [w169] mode=indexing
      tunnel: w44 -> [w170]
      tunnel: [w166] -> w43 mode=indexing
      n85 = Index Array(array=w170, index=w169) -> (element=w168:dbl)
      n86 = Multiply(x=w168, y=200.0) -> (x*y=w166:dbl)
    }
    "Micro-strain" <- w43
    n87 = Not A Number/Path/Refnum?(number/path/refnum=w75) -> (NaN/Path/Refnum?=w144:bool)
    n88 = Less?(x=w75, y=0.0) -> (x < y?=w145:bool)
    n89 = Or(x=w144, y=w145) -> (x .or. y?=w142:bool)
    n90 = property on="RPM_DRVLN_6602" class="DigNum (strict)"("Blinking"=w142) -> ()  [unwired: 2 in, 2 out]
    n91 = Divide(x=w120, y=60.0) -> ()  [unwired: 1 out]
    n92 = Insert Into Array(array=w66, new element=w65) -> (w64:waveform(dbl)[])  [unwired: 1 in]
    n93 = Insert Into Array(array=w64, new element=w61) -> (w63:waveform(dbl)[])  [unwired: 1 in]
    n94 = Insert Into Array(array=w63, new element=w60) -> (w62:waveform(dbl)[])  [unwired: 1 in]
    "Waveform Chart" <- w62
    n95 = disable-structure shown="Disabled" {
      frame Disabled {
        # "TRQ_2SPD_DRVLN_OT"
        n96 = Divide(y=60.0) -> (x/y=w171:dbl)  [unwired: 1 in]
        n97 = Multiply(x=6.283185307179586, y=w171) -> (x*y=w174:dbl)
        n98 = Multiply(y=w174) -> (x*y=→"Power_IN (W)":dbl)  [unwired: 1 in]
      }
      frame Enabled {
      }
    }
    n99 = disable-structure shown="Disabled" {
      disable-tunnel: _ -> [w201 _]
      frame Disabled {
        # "RPM_2SPD_OT"
        # "TRQ_2SPD_OT Wfm"
        # "RPS"
        n100 = Unbundle By Name() -> ("Y"=w205:dbl[])  [unwired: 1 in]
        n101 = call-poly <vilib>:"Mean.vi"("X"=w205) -> ("mean"=w204:dbl)  [unwired: 1 out]
        "TRQ_2SPD_OT (N·m)" <- w204
        n102 = Divide(x=w201, y=60.0) -> (x/y=w202:dbl)
        n103 = Multiply(x=6.283185307179586, y=w202) -> (x*y=w207:dbl)
        n104 = Multiply(x=w204, y=w207) -> (x*y=→"Power_OT (W)":dbl)
      }
      frame Enabled {
      }
    }
    n105 = Unbundle By Name(w42) -> ("status"=w159:bool)
    n106 = Enqueue Element(queue=w91, element=w62, error in (no error)=w90) -> (queue out=w89:refnum<queue>, error out=w88:errorcluster)  [unwired: 1 in, 1 out]
    n107 = Wait (ms)(milliseconds to wait=u32 5) -> ()  [unwired: 1 out]
    n108 = Or(x=w159, y="stop") -> (x .or. y?=w157:bool)
    "AI Producer Iterations" <- w79
  }
  n109 = while {
    tunnel: w11 -> [w236]
    i -> [w235]
    stop <- w227 stop-if-true
    n110 = Dequeue Element(queue=w236) -> (element=w230:waveform(dbl)[], error out=w228:errorcluster)  [unwired: 2 in, 2 out]
    n111 = call "Select_Waveform_By_Name_rev_160122_A.vi"("Array"=string[] ["DataTag"], "Waveform Array"=w230) -> ("Array 2"=w233:waveform(dbl)[])  [unwired: 9 in]
    n112 = call-poly <vilib>:"Index Waveform Array.vi"("waveform array"=w233) -> ("waveform"=w232:waveform(dbl))  [unwired: 9 in, 1 out]
    n113 = Unbundle By Name(w232) -> ("Y"=w231:dbl[])
    n114 = Index Array(array=w231) -> (element=w229:dbl)  [unwired: 1 in]
    n115 = call "Record Continuous Tags Rev 170821_A.vi"("Run Letter"="Run Letter", "path"="path", "Waveform Array In"=w230, "Force Record"="Force Record", "Main Count"=w235, "Num_Blocks"="Num_Blocks", "Data Tag"=w229) -> ("Record Cmd"=w242:bool, "Recorded Blocks"=→"Recorded Blocks":dbl)  [unwired: 2 in, 1 out]
    "Recording" <- w242
    n116 = call <vilib>:"Boolean Crossing PtByPt.vi"("direction"=enum16{"either", "false-true", "true-false"}."true-false", "input"=w242) -> ("crossing"=w243:bool)  [unwired: 1 in]
    n117 = case shown="True" w243 {
      frame False {
      }
      frame True {
        n118 = local write "Data Tag"(99.0 ("y")) -> ()
      }
    }
    n119 = Unbundle By Name(w228) -> ("status"=w227:bool)
    "AI Consumer Iterations" <- w235
  }
  n120 = call <vilib>:"DAQmx Stop Task.vi"("task/channels in"=w18, "error in"=w17) -> ("task out"=w20:refnum<k21>, "error out"=w19:errorcluster)  [unwired: 12 in]
  n121 = Release Queue(queue=w13, error in (no error)=w12) -> ()  [unwired: 1 in, 3 out]
  n122 = call <vilib>:"DAQmx Clear Task.vi"("task in"=w20, "error in"=w19) -> ("error out"=w22:errorcluster)  [unwired: 13 in]
  n123 = call <vilib>:"DAQmx Clear Task.vi"("task in"=w35, "error in"=w3) -> ("error out"=w38:errorcluster)  [unwired: 13 in]
  n124 = call <vilib>:"Simple Error Handler.vi"("type of dialog (OK msg:1)"=w21, "error in (no error)"=w22) -> ()  [unwired: 3 in, 5 out]
  n125 = call <vilib>:"Simple Error Handler.vi"("type of dialog (OK msg:1)"=w33, "error in (no error)"=w38) -> ()  [unwired: 3 in, 5 out]
